vi "test Boolean Data Integrity.vi"(8 "error in (no error)":errorcluster, 11 "Data Manipulation Tests in":refnum<class "Data Manipulation Tests.lvclass">) -> (0 "error out":errorcluster, 3 "Data Manipulation Tests out":refnum<class "Data Manipulation Tests.lvclass">)   [LabVIEW 2017, in "Memory Manager Tests.lvlib" / "Data Manipulation Tests.lvclass"]
uses:
  Data Manipulation Tests.lvclass
  Source/Classes/Pointer/Write Bool.vi
  Source/Classes/Pointer/Write 1D Bool.vi
  Source/Classes/Pointer/Pointer.lvclass
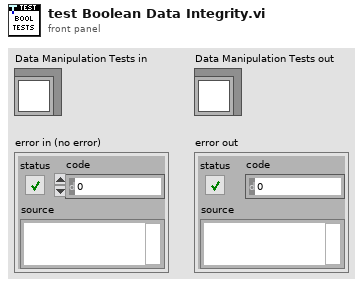
[diagram p1: front panel]
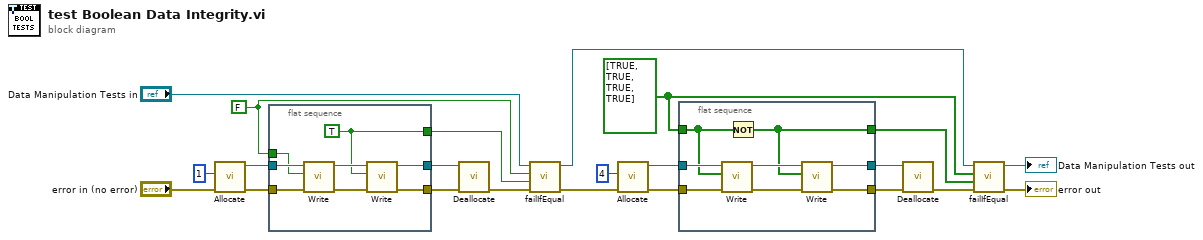
[diagram p0: block diagram]
diagram:
  w16 = bool[] [TRUE, TRUE, TRUE, TRUE] ("value")
  w9 = FALSE ("value")
  n1 = call "Allocate.vi"("error in (no error)"="error in (no error)", "size"=u64 1) -> ("error out"=w6:errorcluster, "Pointer out"=w3:refnum<class "Pointer.lvclass">)  [unwired: 8 in]
  n2 = flat-sequence {
    tunnel: w3 -> [w30]
    tunnel: [w28] -> w4
    tunnel: [w27] -> w5
    tunnel: w6 -> [w25]
    tunnel: w9 -> [w24]
    tunnel: [w23] -> w10
    frame #0 {
      w23 = TRUE ("value")
      n3 = call-poly "Write.vi"("error in (no error)"=w25, "value"=w24, "Pointer in"=w30) -> ("error out"=w26:errorcluster, "Pointer out"=w29:refnum<class "Pointer.lvclass">)  [unwired: 5 in, 2 out]
      n4 = call-poly "Write.vi"("error in (no error)"=w26, "value"=w23, "Pointer in"=w29) -> ("error out"=w27:errorcluster, "Pointer out"=w28:refnum<class "Pointer.lvclass">)  [unwired: 5 in, 2 out]
    }
  }
  n5 = call "Deallocate.vi"("error in (no error)"=w5, "Pointer"=w4) -> ("error out"=w7:errorcluster)  [unwired: 8 in, 1 out]
  n6 = call-dynamic "failIfEqual.vi"("error in (no error)"=w7, "y"=w10, "x"=w9, "TestCase in"="Data Manipulation Tests in") -> ("error out"=w20:errorcluster, "TestCase out"=w19:refnum<class "Data Manipulation Tests.lvclass">)  [unwired: 6 in]
  n7 = call "Allocate.vi"("error in (no error)"=w20, "size"=u64 4) -> ("error out"=w14:errorcluster, "Pointer out"=w11:refnum<class "Pointer.lvclass">)  [unwired: 8 in]
  n8 = flat-sequence {
    tunnel: w11 -> [w38]
    tunnel: [w36] -> w12
    tunnel: [w35] -> w13
    tunnel: w14 -> [w33]
    tunnel: w16 -> [w32]
    tunnel: [w31] -> w17
    frame #0 {
      n9 = call-poly "Write.vi"("error in (no error)"=w33, "buffer in"=w32, "Pointer in"=w38) -> ("error out"=w34:errorcluster, "Pointer out"=w37:refnum<class "Pointer.lvclass">)  [unwired: 5 in, 2 out]
      n10 = Not(x=w32) -> (.not. x?=w31:bool[])
      n11 = call-poly "Write.vi"("error in (no error)"=w34, "buffer in"=w31, "Pointer in"=w37) -> ("error out"=w35:errorcluster, "Pointer out"=w36:refnum<class "Pointer.lvclass">)  [unwired: 5 in, 2 out]
    }
  }
  n12 = call "Deallocate.vi"("error in (no error)"=w13, "Pointer"=w12) -> ("error out"=w15:errorcluster)  [unwired: 8 in, 1 out]
  n13 = call-dynamic "failIfEqual.vi"("error in (no error)"=w15, "y"=w17, "x"=w16, "TestCase in"=w19) -> ("error out"=→"error out":errorcluster, "TestCase out"=→"Data Manipulation Tests out":refnum<class "Data Manipulation Tests.lvclass">)  [unwired: 6 in]
